vi "Redis@HeartBeat__Parameter.vi"(1 "ParamterIn":string) -> (0 "ParamterOut":string)   [LabVIEW 2020]
panel:
  in  "Message=":string
  in  "TimeOut=":string(combo)
  in  "Variable=":string(combo)
  in  "Section":string(combo)
  in  "Value":string
  in  "RedisSession":string(combo)
  in  "Confirm":bool
  # "RedisSession,(Value,Variable=,TimeOut=XXX, Message=XXX)"
  # "@"
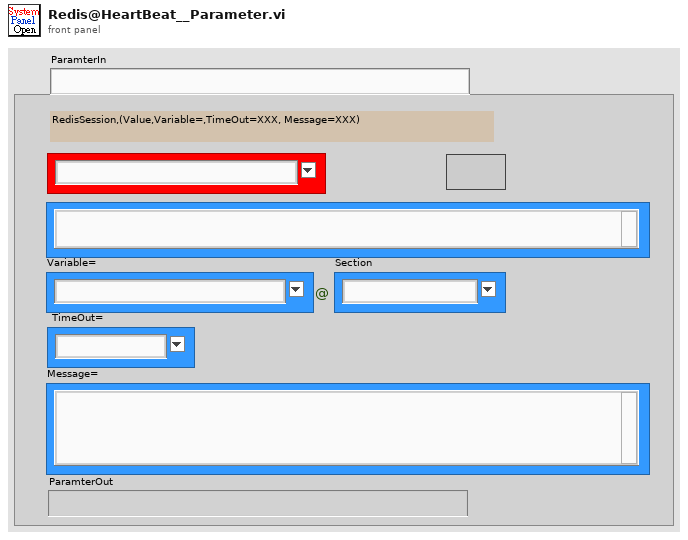
[diagram p1: front panel]
types:
  T1 = enum16{"Get", "Init", "Set", "Delete", "GetElement", "Inc", "Dec"}
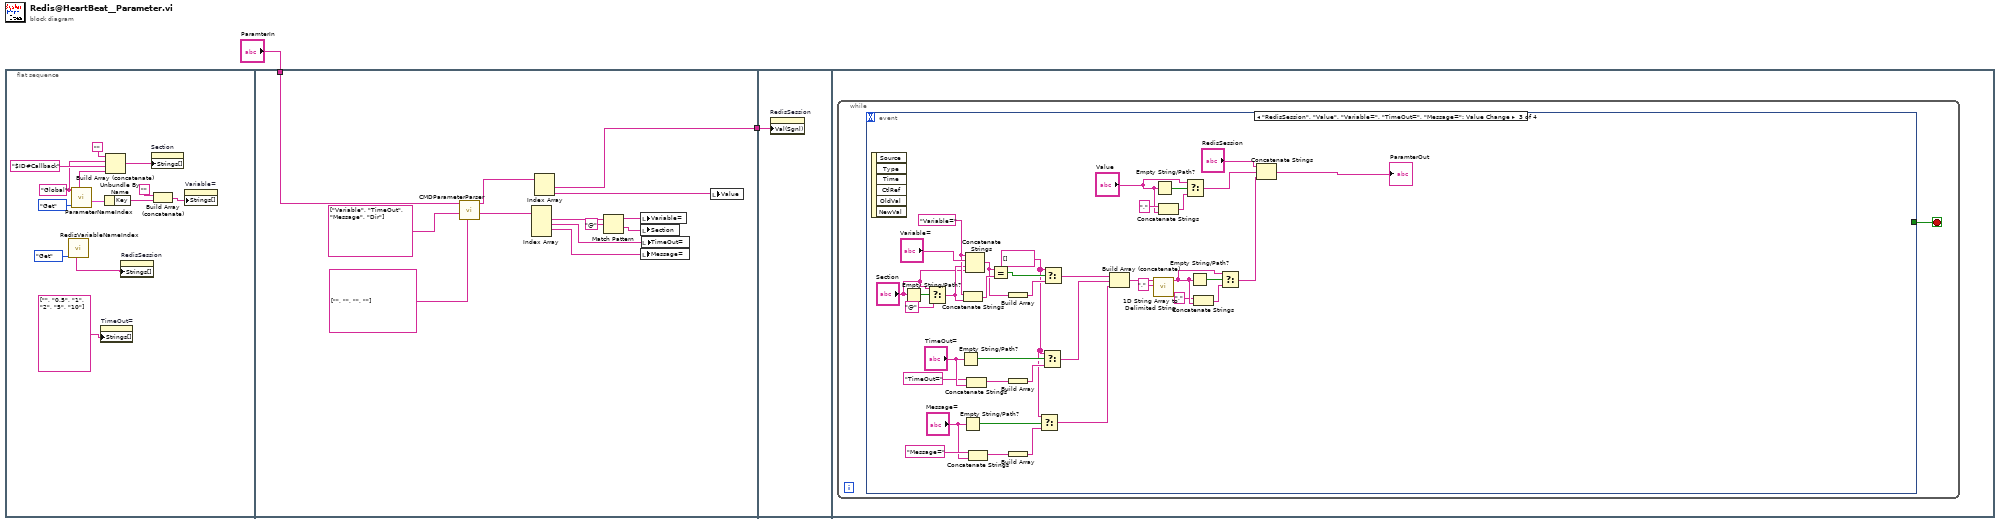
[diagram p0: block diagram]
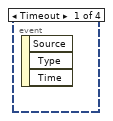
[diagram p2: hidden frame]
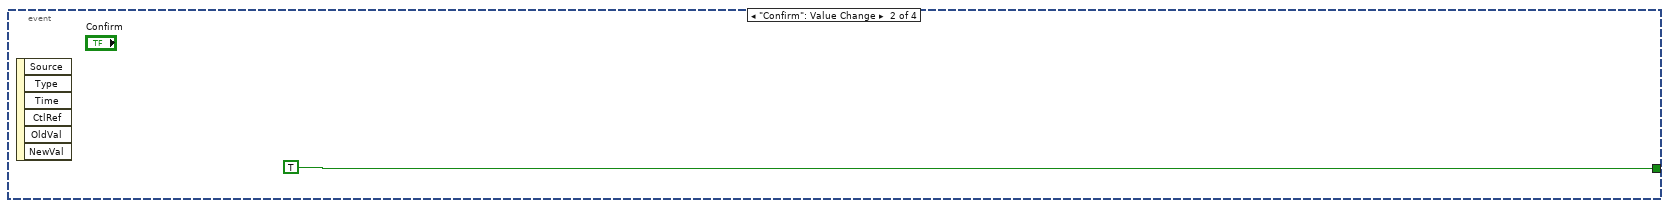
[diagram p3: hidden frame]
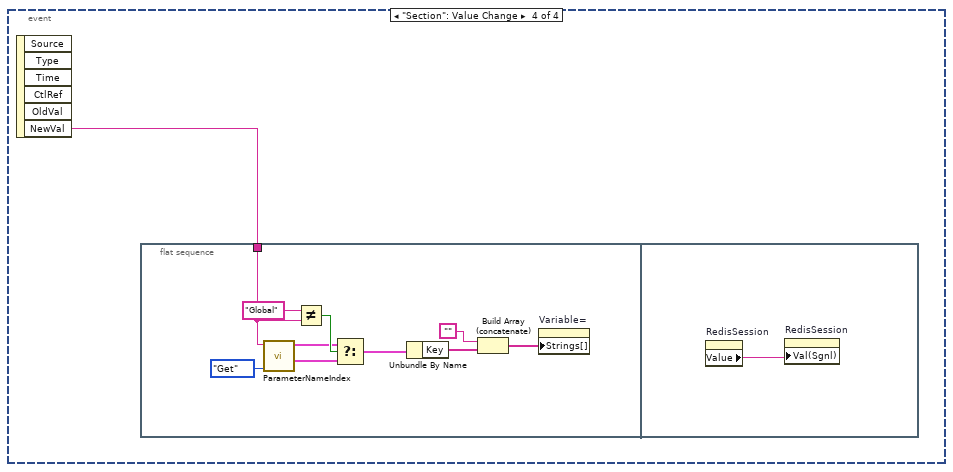
[diagram p4: hidden frame]
diagram:
  n1 = flat-sequence {
    tunnel: "ParamterIn" -> [w28]
    tunnel: [w24] -> w1
    tunnel: w1 -> [w29]
    frame #0 {
      w6 = "Global" ("VariableSection")
      n2 = call "RedisVariableNameIndex.vi"("OP"=enum16{"Add", "Init", "Get"}."Get") -> ("RedisSessionS"=w8:string[])  [unwired: 6 in, 4 out]
      n3 = call "ParameterNameIndex.vi"("OP"=T1."Get", "VariableSection"=w6) -> ("GlobalKeyValue"=w7:cluster{"Key":string[], "Value":string[]}, "SectionList"=w14:string[])  [unwired: 3 in, 5 out]
      n4 = property on="TimeOut=" class="CmbBox"("Strings[]"=string[] ["", "0.5", "1", "2", "5", "10"] ("Strings []")) -> ()  [unwired: 2 in, 2 out]
      n5 = Unbundle By Name(w7) -> ("Key"=w4:string[])
      n6 = Build Array (concatenate)("", w6, "$ID#Callback" ("VariableSection"), w14) -> (w13:string[])
      n7 = property on="RedisSession" class="CmbBox"("Strings[]"=w8) -> ()  [unwired: 2 in, 2 out]
      n8 = property on="Section" class="CmbBox"("Strings[]"=w13) -> ()  [unwired: 2 in, 2 out]
      n9 = Build Array (concatenate)("", w4) -> (w3:string[])
      n10 = property on="Variable=" class="CmbBox"("Strings[]"=w3) -> ()  [unwired: 2 in, 2 out]
    }
    frame #1 {
      n11 = call "CMDParameterParser.vi"("DeafultValues"=string[] ["", "", "", ""], "RequiredKeys"=string[] ["Variable", "TimeOut", "Message", "Dir"], "CMDParameter"=w28) -> ("KeyValues"=w22:string[], "Input"=w25:string[])  [unwired: 6 in, 1 out]
      n12 = Index Array(array=w22) -> (element #1=w21:string, element #2=w18:string, element #3=w17:string)  [unwired: 4 in, 1 out]
      n13 = Index Array(array=w25) -> (element #1=w24:string, element #2=w23:string)  [unwired: 2 in]
      n14 = Match Pattern(string=w21, regular expression="@") -> (before substring=w19:string, after substring=w16:string)  [unwired: 1 in, 2 out]
      n15 = local write "Variable="(w19) -> ()
      n16 = local write "Section"(w16) -> ()
      n17 = local write "Message="(w17) -> ()
      n18 = local write "TimeOut="(w18) -> ()
      n19 = local write "Value"(w23) -> ()
    }
    frame #2 {
      n20 = property on="RedisSession" class="CmbBox"("Val(Sgnl)"=w29) -> ()  [unwired: 2 in, 2 out]
    }
    frame #3 {
      n21 = while {
        stop <- w30 stop-if-true
        n22 = event shown="[2] \"RedisSession\", \"Value\", \"Variable=\", \"TimeOut=\", \"Message=\": Value Change" {
          selector: _ -> [_ _ _ _]
          dyn-events: _ -> [_ _ _ _]
          timeout: _ -> [_ _ _ _]
          tunnel: [_ TRUE _ _] -> w30
          event Timeout {
            n23 = event-data() -> ()  [unwired: 1 in, 3 out]
          }
          event "Confirm": Value Change {
            n24 = event-data() -> ()  [unwired: 1 in, 6 out]
          }
          event "RedisSession", "Value", "Variable=", "TimeOut=", "Message=": Value Change {
            w52 = string[] [] ("t")
            w65 = "Variable=" ("string")
            n25 = event-data() -> ()  [unwired: 1 in, 6 out]
            n26 = Empty String/Path?(string/path="Section") -> (empty?=w40:bool)
            n27 = Select(t="Section", s=w40, f="@") -> (s? t:f=w38:string)
            n28 = Empty String/Path?(string/path="TimeOut=") -> (empty?=w64:bool)
            n29 = Empty String/Path?(string/path="Message=") -> (empty?=w59:bool)
            n30 = Concatenate Strings(w65, w38) -> (w58:string)
            n31 = Concatenate Strings(w65, "Variable=", w38, "Section") -> (w41:string)
            n32 = Concatenate Strings("TimeOut=" ("string"), "TimeOut=") -> (w56:string)
            n33 = Concatenate Strings("Message=" ("string"), "Message=") -> (w54:string)
            n34 = Equal?(x=w41, y=w58) -> (x = y?=w66:bool)
            n35 = Build Array(w41) -> (w57:string[])
            n36 = Build Array(w56) -> (w55:string[])
            n37 = Build Array(w54) -> (w53:string[])
            n38 = Select(t=w52, s=w59, f=w53) -> (s? t:f=w49:string[])
            n39 = Select(t=w52, s=w64, f=w55) -> (s? t:f=w50:string[])
            n40 = Select(t=w52, s=w66, f=w57) -> (s? t:f=w51:string[])
            n41 = Build Array (concatenate)(w51, w50, w49) -> (w48:string[])
            n42 = call <vilib>:"1D String Array to Delimited String.vi"("delimiter"=",", "string array"=w48) -> ("delimited string"=w45:string)  [unwired: 9 in]
            n43 = Empty String/Path?(string/path="Value") -> (empty?=w34:bool)
            n44 = Concatenate Strings("," ("string"), "Value") -> (w36:string)
            n45 = Select(t="Value", s=w34, f=w36) -> (s? t:f=w32:string)
            n46 = Empty String/Path?(string/path=w45) -> (empty?=w46:bool)
            n47 = Concatenate Strings("," ("string"), w45) -> (w43:string)
            n48 = Select(t=w45, s=w46, f=w43) -> (s? t:f=w42:string)
            n49 = Concatenate Strings("RedisSession", w32, w42) -> (→"ParamterOut":string)
          }
          event "Section": Value Change {
            n50 = event-data() -> ("NewVal"=w70:string)  [unwired: 1 in, 5 out]
            n51 = flat-sequence {
              tunnel: w70 -> [w79]
              frame #0 {
                n52 = call "ParameterNameIndex.vi"("OP"=T1."Get", "VariableSection"=w79) -> ("GlobalKeyValue"=w75:cluster{"Key":string[], "Value":string[]}, "SectionKeyValue"=w76:cluster{"Key":string[], "Value":string[]})  [unwired: 3 in, 5 out]
                n53 = Not Equal?(x="Global", y=w79) -> (x != y?=w77:bool)
                n54 = Select(t=w76, s=w77, f=w75) -> (s? t:f=w74:cluster{"Key":string[], "Value":string[]})
                n55 = Unbundle By Name(w74) -> ("Key"=w73:string[])
                n56 = Build Array (concatenate)("", w73) -> (w71:string[])
                n57 = property on="Variable=" class="CmbBox"("Strings[]"=w71) -> ()  [unwired: 2 in, 2 out]
              }
              frame #1 {
                n58 = property on="RedisSession" class="CmbBox"() -> ("Value"=w81:string)  [unwired: 2 in, 2 out]
                n59 = property on="RedisSession" class="CmbBox"("Val(Sgnl)"=w81) -> ()  [unwired: 2 in, 2 out]
              }
            }
          }
        }
      }
    }
  }
